vi "压装试验判定.vi"(7 "Result":refnum<vi>, 10 "判定参数":T1, 11 "XY曲线":cluster{"X":dbl[], "Y":dbl[]}[](array[cluster])) -> (2 "判定项长度":i32, 3 "OK？":bool)   [LabVIEW 2020]
panel:
  out "第二段":dbl
  out "第一段":dbl
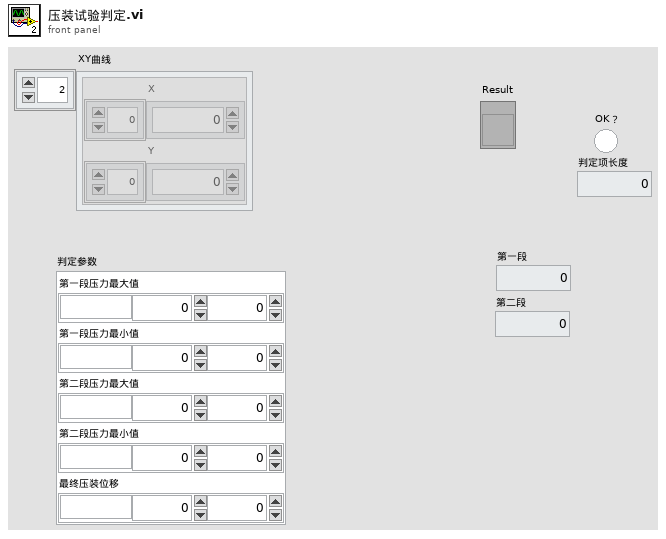
[diagram p1: front panel]
types:
  T1 = cluster{"第一段压力最大值":cluster{"单位":string, "下限":dbl, "上限":dbl}, "第一段压力最小值":cluster{"单位":string, "下限":dbl, "上限":dbl}, "第二段压力最大值":cluster{"单位":string, "下限":dbl, "上限":dbl}, "第二段压力最小值":cluster{"单位":string, "下限":dbl, "上限":dbl}, "最终压装位移":cluster{"单位":string, "下限":dbl, "上限":dbl}}
  T2 = cluster{"第一段位移":cluster{"单位":string, "下限":dbl, "上限":dbl}, "第一段压力":cluster{"单位":string, "下限":dbl, "上限":dbl}, "第二段位移":cluster{"单位":string, "下限":dbl, "上限":dbl}, "第二段压力":cluster{"单位":string, "下限":dbl, "上限":dbl}}
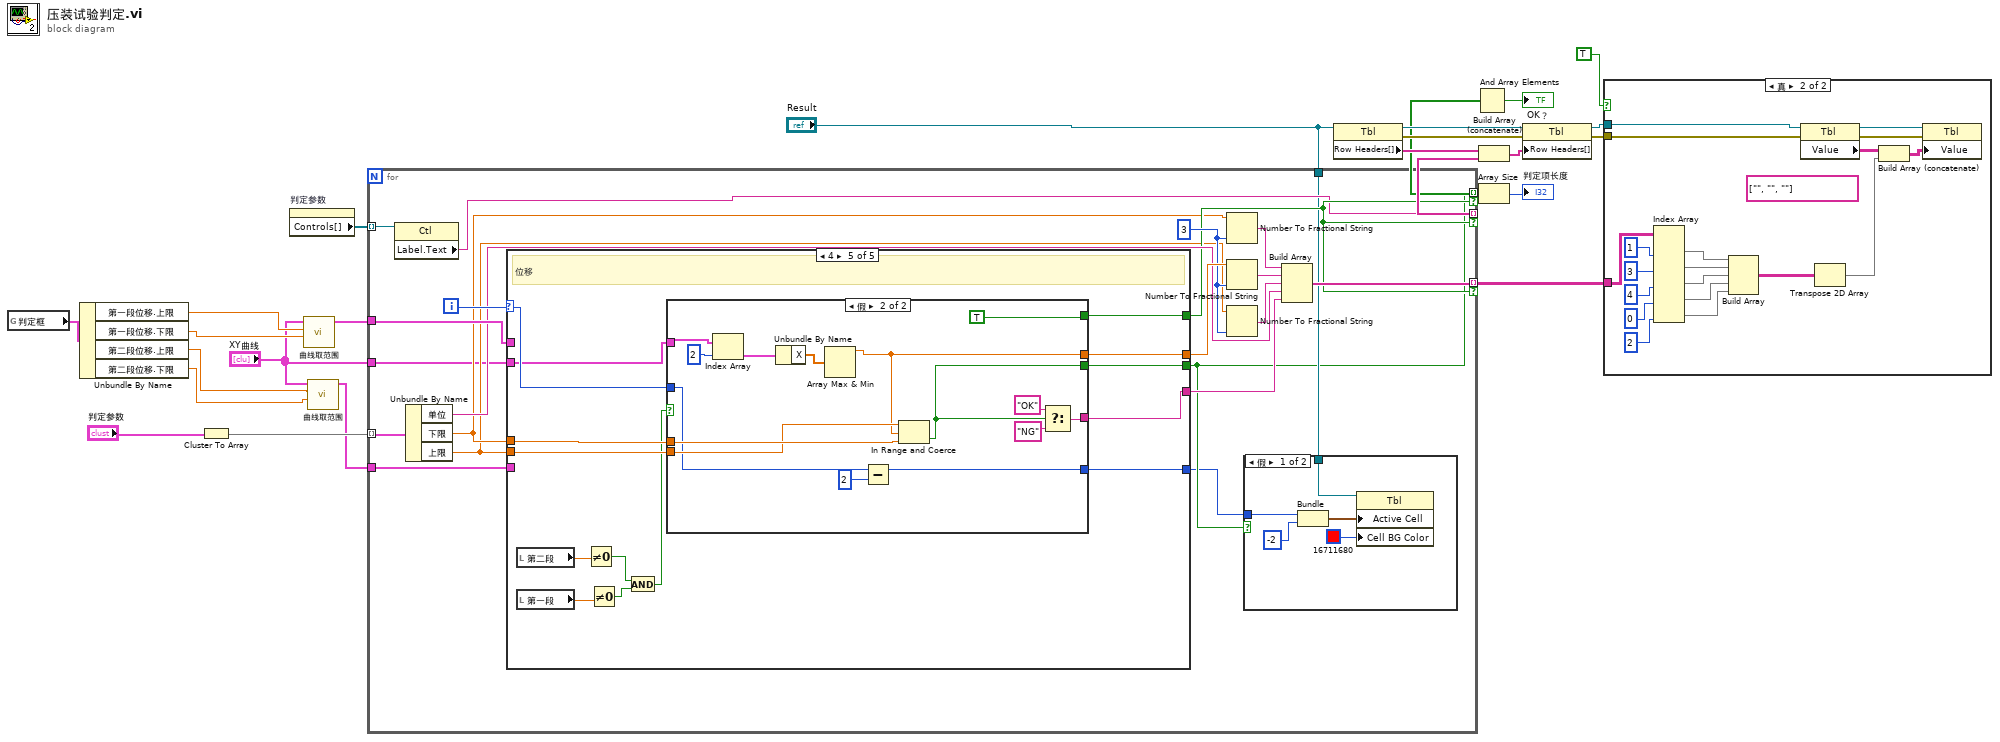
[diagram p0: block diagram]
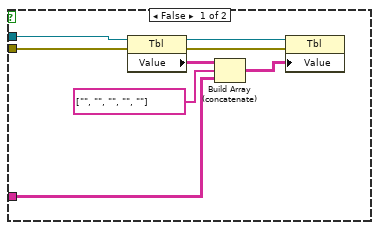
[diagram p2: hidden frame]
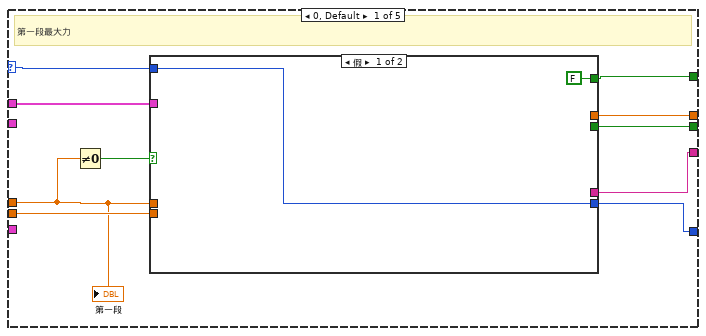
[diagram p4: hidden frame]
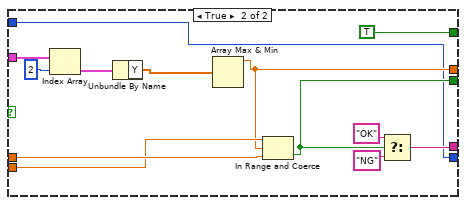
[diagram p5: hidden frame]
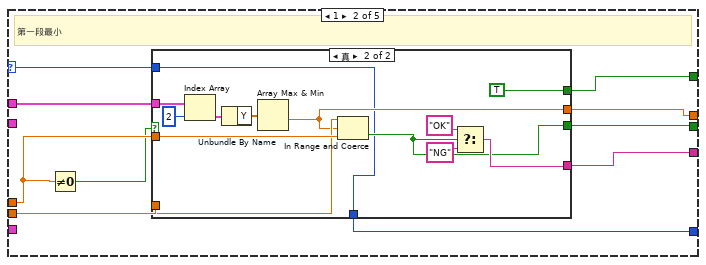
[diagram p6: hidden frame]
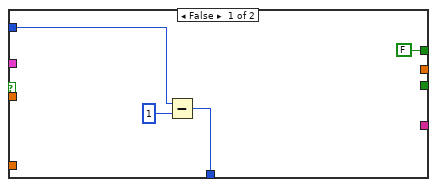
[diagram p7: hidden frame]
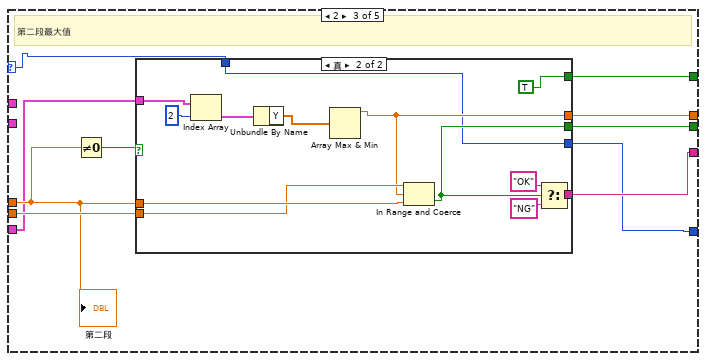
[diagram p8: hidden frame]
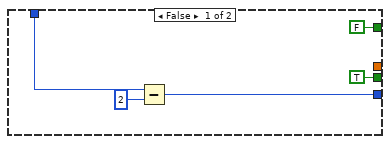
[diagram p9: hidden frame]
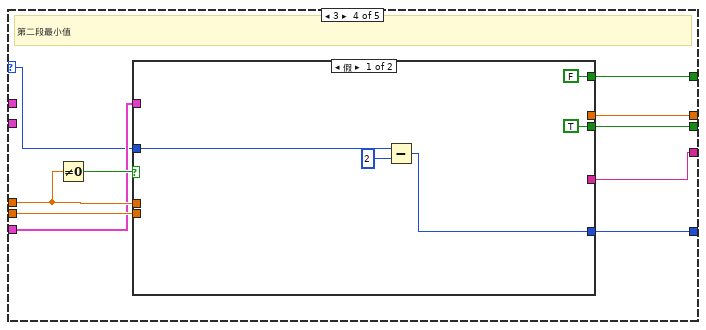
[diagram p10: hidden frame]
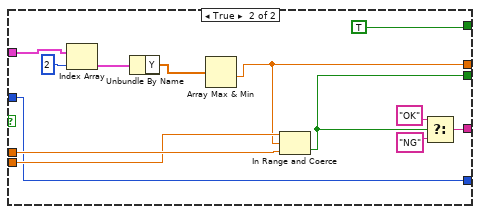
[diagram p11: hidden frame]
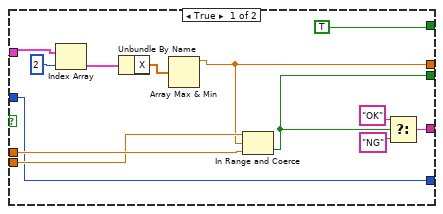
[diagram p12: hidden frame]
diagram:
  n1 = global read "判定参数.vi" "判定框"() -> (w6:T2)
  n2 = Unbundle By Name(w6) -> ("第一段位移.上限"=w8:dbl, "第一段位移.下限"=w7:dbl, "第二段位移.上限"=w3:dbl, "第二段位移.下限"=w2:dbl)
  n3 = Cluster To Array(cluster="判定参数") -> (array=w24:cluster{"单位":string, "下限":dbl, "上限":dbl}[])
  n4 = property on="判定参数" class="Clust (严格)"() -> ("Controls[]"=w14:refnum<vi>[])  [unwired: 2 in, 2 out]
  n5 = call "曲线取范围.vi"("下限"=w7, "上限"=w8, "曲线In"="XY曲线") -> ("曲线Out"=w10:cluster{"X":dbl[], "Y":dbl[]}[])  [unwired: 8 in]
  n6 = call "曲线取范围.vi"("下限"=w2, "上限"=w3, "曲线In"="XY曲线") -> ("曲线Out"=w5:cluster{"X":dbl[], "Y":dbl[]}[])  [unwired: 8 in]
  n7 = for {
    tunnel: w24 -> [w45] mode=indexing
    tunnel: w14 -> [w43] mode=indexing
    tunnel: w10 -> [w41]
    tunnel: [w27] -> w12 mode=indexing if=w33
    tunnel: [w34] -> w15 mode=indexing if=w33
    tunnel: [w30] -> w17 mode=indexing if=w33
    tunnel: w5 -> [w29]
    tunnel: "Result" -> [w28]
    tunnel: "XY曲线" -> [w25]
    i -> [w44]
    w40 = i16 3 ("精度(6)")
    n8 = property class="Ctl"(reference=w43) -> ("Label.Text"=w30:string)  [unwired: 1 in, 2 out]
    n9 = Unbundle By Name(w45) -> ("单位"=w35:string, "下限"=w32:dbl, "上限"=w31:dbl)
    n10 = case shown="4" w44 {
      selector: w44 -> [w51 w77 w104 w132 w166]
      tunnel: [w55 w80 w109 w136 w168] -> w42
      tunnel: w41 -> [w60 w85 _ _ _]
      tunnel: [w59 w84 w112 w140 w172] -> w36
      tunnel: [w58 w83 w111 w139 w171] -> w27
      tunnel: w32 -> [w53 w79 w108 w135 w167]
      tunnel: w31 -> [w57 w82 w110 w138 w170]
      tunnel: [w56 w81 w106 w137 w169] -> w33
      tunnel: w29 -> [_ _ w105 w133 _]
      tunnel: [w52 w76 w103 w131 w165] -> w26
      tunnel: w25 -> [_ _ _ _ w159]
      frame 0, Default {
        # "第一段最大力"
        n11 = Not Equal To 0?(x=w53) -> (x != 0?=w54:bool)
        n12 = case shown="假" w54 {
          tunnel: w60 -> [_ w75]
          tunnel: [_ w70] -> w59
          tunnel: [_ w69] -> w58
          tunnel: w53 -> [_ w68]
          tunnel: w57 -> [_ w67]
          tunnel: [FALSE TRUE] -> w56
          tunnel: [_ w64] -> w55
          tunnel: [w61 w63] -> w52
          tunnel: w51 -> [w61 w63]
          frame False {
          }
          frame True {
            n13 = Index Array(array=w75, index=2 ("索引")) -> (element=w73:cluster{"X":dbl[], "Y":dbl[]})
            n14 = Unbundle By Name(w73) -> ("Y"=w65:dbl[])
            n15 = Array Max & Min(array=w65) -> (max value=w64:dbl)  [unwired: 3 out]
            n16 = In Range and Coerce(upper limit=w67, x=w64, lower limit=w68) -> (In Range?=w69:bool)  [unwired: 1 out]
            n17 = Select(t="OK", s=w69, f="NG") -> (s? t:f=w70:string)
          }
        }
        "第一段" <- w53
      }
      frame 1 {
        # "第一段最小"
        n18 = Not Equal To 0?(x=w79) -> (x != 0?=w78:bool)
        n19 = case shown="真" w78 {
          tunnel: w85 -> [_ w102]
          tunnel: [_ w98] -> w84
          tunnel: [_ w97] -> w83
          tunnel: w79 -> [_ w96]
          tunnel: w82 -> [_ w95]
          tunnel: [FALSE TRUE] -> w81
          tunnel: [_ w91] -> w80
          tunnel: w77 -> [w88 w90]
          tunnel: [w87 w90] -> w76
          frame False {
            n20 = Subtract(x=w88, y=1) -> (x-y=w87:i32)
          }
          frame True {
            n21 = Index Array(array=w102, index=2 ("索引")) -> (element=w101:cluster{"X":dbl[], "Y":dbl[]})
            n22 = Unbundle By Name(w101) -> ("Y"=w93:dbl[])
            n23 = Array Max & Min(array=w93) -> (min value=w91:dbl)  [unwired: 3 out]
            n24 = In Range and Coerce(upper limit=w95, x=w91, lower limit=w96) -> (In Range?=w97:bool)  [unwired: 1 out]
            n25 = Select(t="OK", s=w97, f="NG") -> (s? t:f=w98:string)
          }
        }
      }
      frame 2 {
        # "第二段最大值"
        n26 = Not Equal To 0?(x=w108) -> (x != 0?=w107:bool)
        n27 = case shown="真" w107 {
          tunnel: [_ w127] -> w112
          tunnel: [TRUE w126] -> w111
          tunnel: w108 -> [_ w125]
          tunnel: w110 -> [_ w124]
          tunnel: [_ w121] -> w109
          tunnel: w105 -> [_ w120]
          tunnel: [FALSE TRUE] -> w106
          tunnel: w104 -> [w115 w118]
          tunnel: [w114 w118] -> w103
          frame False {
            n28 = Subtract(x=w115, y=2) -> (x-y=w114:i32)
          }
          frame True {
            n29 = Index Array(array=w120, index=2 ("索引")) -> (element=w123:cluster{"X":dbl[], "Y":dbl[]})
            n30 = Unbundle By Name(w123) -> ("Y"=w122:dbl[])
            n31 = Array Max & Min(array=w122) -> (max value=w121:dbl)  [unwired: 3 out]
            n32 = In Range and Coerce(upper limit=w124, x=w121, lower limit=w125) -> (In Range?=w126:bool)  [unwired: 1 out]
            n33 = Select(t="OK", s=w126, f="NG") -> (s? t:f=w127:string)
          }
        }
        "第二段" <- w108
      }
      frame 3 {
        # "第二段最小值"
        n34 = Not Equal To 0?(x=w135) -> (x != 0?=w134:bool)
        n35 = case shown="假" w134 {
          tunnel: [_ w155] -> w140
          tunnel: [TRUE w154] -> w139
          tunnel: w135 -> [_ w153]
          tunnel: w138 -> [_ w152]
          tunnel: [FALSE TRUE] -> w137
          tunnel: [_ w148] -> w136
          tunnel: w133 -> [_ w147]
          tunnel: w132 -> [w143 w146]
          tunnel: [w142 w146] -> w131
          frame False {
            n36 = Subtract(x=w143, y=2) -> (x-y=w142:i32)
          }
          frame True {
            n37 = Index Array(array=w147, index=2 ("索引")) -> (element=w150:cluster{"X":dbl[], "Y":dbl[]})
            n38 = Unbundle By Name(w150) -> ("Y"=w149:dbl[])
            n39 = Array Max & Min(array=w149) -> (min value=w148:dbl)  [unwired: 3 out]
            n40 = In Range and Coerce(upper limit=w152, x=w148, lower limit=w153) -> (In Range?=w154:bool)  [unwired: 1 out]
            n41 = Select(t="OK", s=w154, f="NG") -> (s? t:f=w155:string)
          }
        }
      }
      frame 4 {
        # "位移"
        n42 = local read "第二段"() -> (w164:dbl)
        n43 = local read "第一段"() -> (w163:dbl)
        n44 = Not Equal To 0?(x=w164) -> (x != 0?=w161:bool)
        n45 = Not Equal To 0?(x=w163) -> (x != 0?=w162:bool)
        n46 = And(x=w161, y=w162) -> (x .and. y?=w160:bool)
        n47 = case shown="假" w160 {
          tunnel: [w182 w197] -> w172
          tunnel: [w181 w196] -> w171
          tunnel: w167 -> [w180 w195]
          tunnel: w170 -> [w179 w194]
          tunnel: [TRUE TRUE] -> w169
          tunnel: [w174 w189] -> w168
          tunnel: w159 -> [w175 w190]
          tunnel: w166 -> [w173 w188]
          tunnel: [w173 w187] -> w165
          frame True {
            n48 = Index Array(array=w175, index=2 ("索引")) -> (element=w177:cluster{"X":dbl[], "Y":dbl[]})
            n49 = Unbundle By Name(w177) -> ("X"=w176:dbl[])
            n50 = Array Max & Min(array=w176) -> (max value=w174:dbl)  [unwired: 3 out]
            n51 = In Range and Coerce(upper limit=w179, x=w174, lower limit=w180) -> (In Range?=w181:bool)  [unwired: 1 out]
            n52 = Select(t="OK", s=w181, f="NG") -> (s? t:f=w182:string)
          }
          frame False {
            n53 = Index Array(array=w190, index=2 ("索引")) -> (element=w192:cluster{"X":dbl[], "Y":dbl[]})
            n54 = Unbundle By Name(w192) -> ("X"=w191:dbl[])
            n55 = Array Max & Min(array=w191) -> (max value=w189:dbl)  [unwired: 3 out]
            n56 = Subtract(x=w188, y=2) -> (x-y=w187:i32)
            n57 = In Range and Coerce(upper limit=w194, x=w189, lower limit=w195) -> (In Range?=w196:bool)  [unwired: 1 out]
            n58 = Select(t="OK", s=w196, f="NG") -> (s? t:f=w197:string)
          }
        }
      }
    }
    n59 = Number To Fractional String(number=w32, precision (6)=w40) -> (F-format string=w39:string)  [unwired: 2 in]
    n60 = Number To Fractional String(number=w42, precision (6)=w40) -> (F-format string=w38:string)  [unwired: 2 in]
    n61 = Number To Fractional String(number=w31, precision (6)=w40) -> (F-format string=w37:string)  [unwired: 2 in]
    n62 = case shown="假" w27 {
      tunnel: w28 -> [w50 _]
      tunnel: w26 -> [w46 _]
      frame False {
        n63 = Bundle(w46, "索引"=-2) -> (w47:cluster{i32, "索引":i32})  [unwired: 1 in]
        n64 = property class="Tbl"(reference=w50, "Active Cell"=w47, "Cell BG Color"=u32 16711680 ("活动单元格:单元格背景色")) -> ()  [unwired: 1 in, 2 out]
      }
      frame True {
      }
    }
    n65 = Build Array(w39, w38, w37, w35, w36) -> (w34:string[])
  }
  n66 = property class="Tbl"(reference="Result") -> (reference out=w19:refnum<vi>, error out=w22:errorcluster, "Row Headers[]"=w16:string[])  [unwired: 1 in]
  n67 = And Array Elements(Boolean array=w12) -> (logical AND=→"OK？":bool)
  n68 = Build Array (concatenate)(w16, w17) -> (w18:string[])
  n69 = Array Size(array=w12) -> (size(s)=→"判定项长度":i32)
  n70 = property class="Tbl"(reference=w19, error in=w22, "Row Headers[]"=w18) -> (reference out=w20:refnum<vi>, error out=w21:errorcluster)
  n71 = case shown="真" TRUE {
    tunnel: w21 -> [w206 w225]
    tunnel: w20 -> [w203 w222]
    tunnel: w15 -> [w202 w221]
    frame False {
      n72 = property class="Tbl"(reference=w203, error in=w206) -> (reference out=w204:refnum<vi>, error out=w205:errorcluster, "Value"=w207:string[][])
      n73 = Build Array (concatenate)(w207, string[] ["", "", "", "", ""], w202) -> (w208:string[][])
      n74 = property class="Tbl"(reference=w204, error in=w205, "Value"=w208) -> ()  [unwired: 2 out]
    }
    frame True {
      (unwired) string[] ["", "", ""]
      n75 = Index Array(array=w221, index (col) #1=1 ("禁用的索引 (列)"), index (col) #2=3 ("索引 (列)"), index (col) #3=4 ("索引 (列)"), index (col) #4=0 ("索引 (列)"), index (col) #5=2 ("索引 (列)")) -> (element #1=w217:string[], element #2=w216:string[], element #3=w215:string[], element #4=w210:string[], element #5=w209:string[])  [unwired: 5 in]
      n76 = Build Array(w217, w216, w215, w210, w209) -> (w214:string[][])
      n77 = property class="Tbl"(reference=w222, error in=w225) -> (reference out=w223:refnum<vi>, error out=w224:errorcluster, "Value"=w226:string[][])
      n78 = Transpose 2D Array(2D array=w214) -> (transposed array=w213:string[][])
      n79 = Build Array (concatenate)(w226, w213) -> (w227:string[][])
      n80 = property class="Tbl"(reference=w223, error in=w224, "Value"=w227) -> ()  [unwired: 2 out]
    }
  }
